vi "Brute Force Measurment SubVI.vi"() -> ()   [LabVIEW 2020]
panel:
  out "Boolean array 2":bool[](array[boolean])
  in  "Number of Active tubes":i32
  out "Clear Pin Task Out 2":refnum<k21>
  in  "Clear Pin Task In 2":refnum<k21>
  in  "Sync Pin Task In":refnum<k21>
  out "Sync Pin Task Out":refnum<k21>
  out "Clear Pin Task Out":refnum<k21>
  in  "Clear Pin Task In":refnum<k21>
  out "Boolean array":bool[](array[boolean])
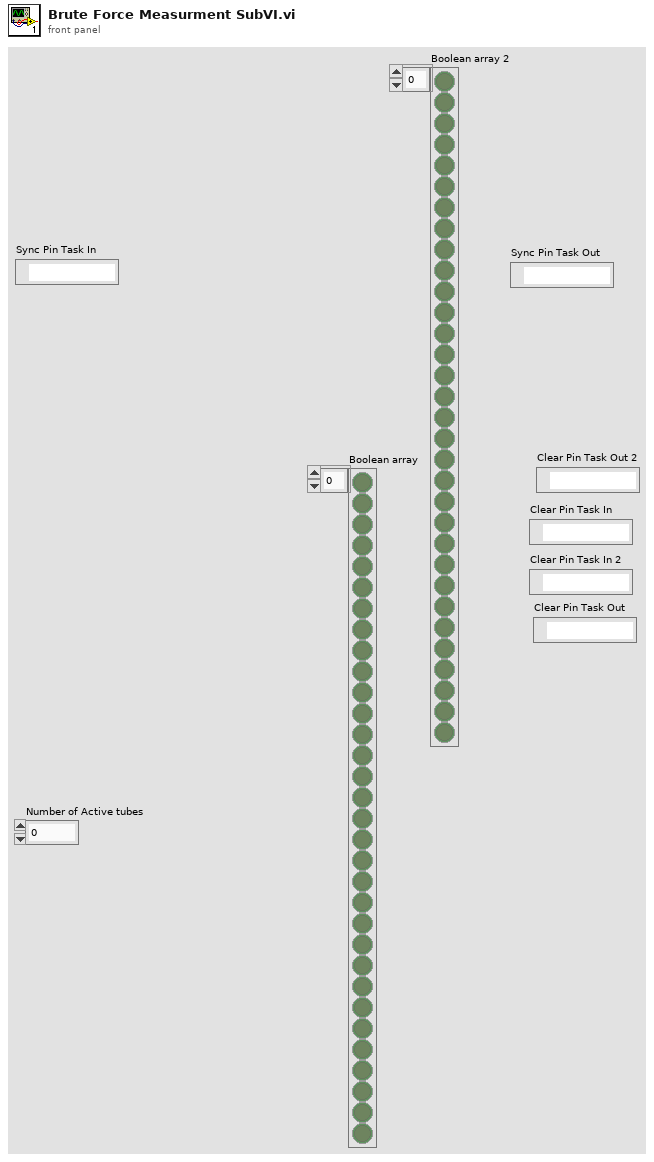
[diagram p1: front panel]
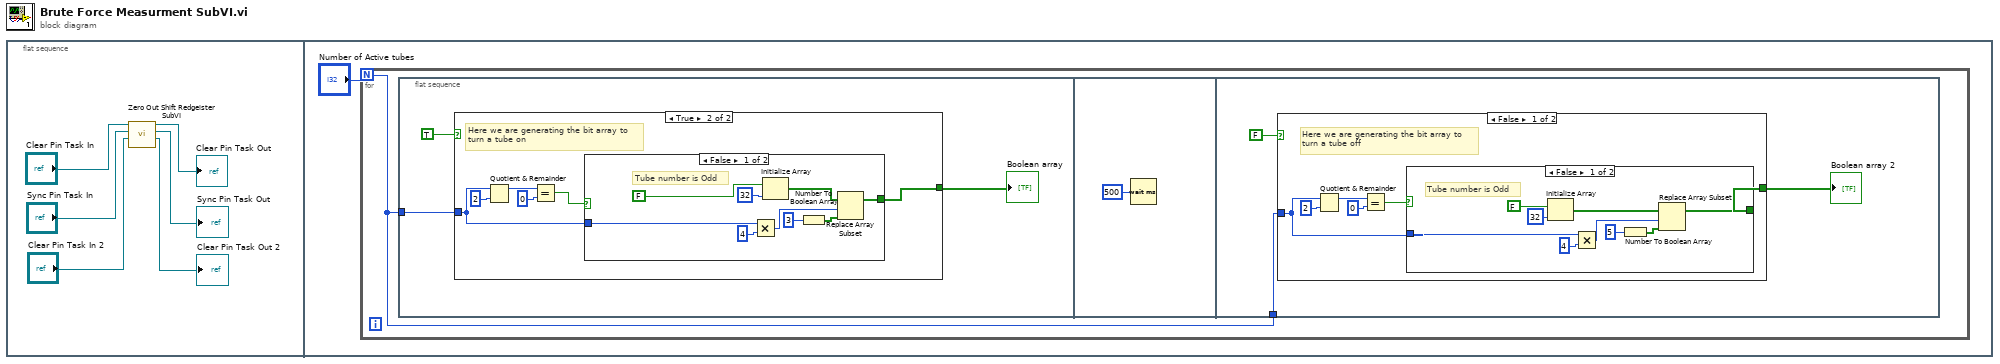
[diagram p0: block diagram]
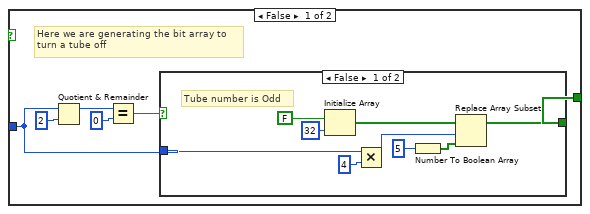
[diagram p2: hidden frame]
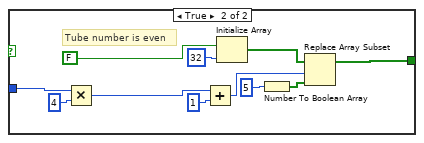
[diagram p3: hidden frame]
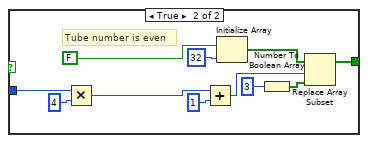
[diagram p4: hidden frame]
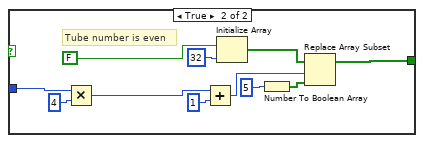
[diagram p5: hidden frame]
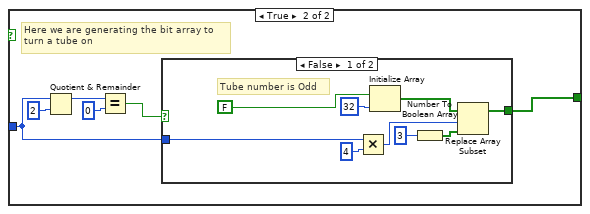
[diagram p6: hidden frame]
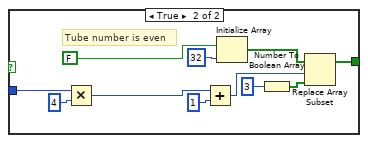
[diagram p7: hidden frame]
diagram:
  n1 = flat-sequence {
    frame #0 {
      n2 = call "Zero Out Shift Redgeister SubVI.vi"("Clear Pin Task In in"="Clear Pin Task In 2", "Sync Pin Task In"="Sync Pin Task In", "Refnum in"="Clear Pin Task In") -> ("Clear Pin Task Out 2"=→"Clear Pin Task Out 2":refnum<k21>, "Sync Pin Task Out"=→"Sync Pin Task Out":refnum<k21>, "Refnum out"=→"Clear Pin Task Out":refnum<k21>)  [unwired: 6 in]
    }
    frame #1 {
      n3 = for {
        N: "Number of Active tubes" -> [w8]
        n4 = flat-sequence {
          tunnel: w8 -> [w10]
          tunnel: w8 -> [w66]
          frame #0 {
            n5 = case shown="True" TRUE {
              tunnel: w10 -> [w13 w42]
              tunnel: [w14 w43] -> w11
              frame False {
                # "Here we are generating the bit array to \nturn a tube off"
                n6 = Quotient & Remainder(x=w13, y=2) -> (x-y*floor(x/y)=w16:i32)  [unwired: 1 out]
                n7 = Equal?(x=w16, y=0) -> (x = y?=w12:bool)
                n8 = case shown="False" w12 {
                  tunnel: w13 -> [w24 w32]
                  tunnel: [w18 w33] -> w14
                  frame False {
                    # "Tube number is Odd"
                    n9 = Initialize Array(FALSE, 32) -> (w20:bool[])
                    n10 = Multiply(x=w24, y=4) -> (x*y=w19:i32)
                    n11 = Number To Boolean Array(number=5) -> (Boolean array=w23:bool[])
                    n12 = Replace Array Subset(array=w20, new element=w23, index=w19) -> (w18:bool[])
                  }
                  frame True {
                    # "Tube number is even"
                    n13 = Multiply(x=w32, y=4) -> (x*y=w28:i32)
                    n14 = Add(x=w28, y=1) -> (x+y=w29:i32)
                    n15 = Initialize Array(FALSE, 32) -> (w35:bool[])
                    n16 = Number To Boolean Array(number=5) -> (Boolean array=w30:bool[])
                    n17 = Replace Array Subset(array=w35, new element=w30, index=w29) -> (w33:bool[])
                  }
                }
              }
              frame True {
                # "Here we are generating the bit array to \nturn a tube on"
                n18 = Quotient & Remainder(x=w42, y=2) -> (x-y*floor(x/y)=w40:i32)  [unwired: 1 out]
                n19 = Equal?(x=w40, y=0) -> (x = y?=w38:bool)
                n20 = case shown="False" w38 {
                  tunnel: w42 -> [w47 w58]
                  tunnel: [w45 w59] -> w43
                  frame False {
                    # "Tube number is Odd"
                    n21 = Multiply(x=w47, y=4) -> (x*y=w46:i32)
                    n22 = Initialize Array(FALSE, 32) -> (w50:bool[])
                    n23 = Number To Boolean Array(number=3) -> (Boolean array=w44:bool[])
                    n24 = Replace Array Subset(array=w50, new element=w44, index=w46) -> (w45:bool[])
                  }
                  frame True {
                    # "Tube number is even"
                    n25 = Multiply(x=w58, y=4) -> (x*y=w54:i32)
                    n26 = Add(x=w54, y=1) -> (x+y=w55:i32)
                    n27 = Initialize Array(FALSE, 32) -> (w61:bool[])
                    n28 = Number To Boolean Array(number=3) -> (Boolean array=w56:bool[])
                    n29 = Replace Array Subset(array=w61, new element=w56, index=w55) -> (w59:bool[])
                  }
                }
              }
            }
            "Boolean array" <- w11
          }
          frame #1 {
            n30 = Wait (ms)(milliseconds to wait=u32 500) -> ()  [unwired: 1 out]
          }
          frame #2 {
            n31 = case shown="False" FALSE {
              tunnel: w66 -> [w69 w98]
              tunnel: [w70 w99] -> w67
              frame False {
                # "Here we are generating the bit array to \nturn a tube off"
                n32 = Quotient & Remainder(x=w69, y=2) -> (x-y*floor(x/y)=w72:i32)  [unwired: 1 out]
                n33 = Equal?(x=w72, y=0) -> (x = y?=w68:bool)
                n34 = case shown="False" w68 {
                  tunnel: w69 -> [w80 w88]
                  tunnel: [w74 w89] -> w70
                  frame False {
                    # "Tube number is Odd"
                    n35 = Initialize Array(FALSE, 32) -> (w76:bool[])
                    n36 = Multiply(x=w80, y=4) -> (x*y=w75:i32)
                    n37 = Number To Boolean Array(number=5) -> (Boolean array=w79:bool[])
                    n38 = Replace Array Subset(array=w76, new element=w79, index=w75) -> (w74:bool[])
                  }
                  frame True {
                    # "Tube number is even"
                    n39 = Multiply(x=w88, y=4) -> (x*y=w84:i32)
                    n40 = Add(x=w84, y=1) -> (x+y=w85:i32)
                    n41 = Initialize Array(FALSE, 32) -> (w91:bool[])
                    n42 = Number To Boolean Array(number=5) -> (Boolean array=w86:bool[])
                    n43 = Replace Array Subset(array=w91, new element=w86, index=w85) -> (w89:bool[])
                  }
                }
              }
              frame True {
                # "Here we are generating the bit array to \nturn a tube on"
                n44 = Quotient & Remainder(x=w98, y=2) -> (x-y*floor(x/y)=w96:i32)  [unwired: 1 out]
                n45 = Equal?(x=w96, y=0) -> (x = y?=w94:bool)
                n46 = case shown="False" w94 {
                  tunnel: w98 -> [w103 w114]
                  tunnel: [w101 w115] -> w99
                  frame False {
                    # "Tube number is Odd"
                    n47 = Multiply(x=w103, y=4) -> (x*y=w102:i32)
                    n48 = Initialize Array(FALSE, 32) -> (w106:bool[])
                    n49 = Number To Boolean Array(number=3) -> (Boolean array=w100:bool[])
                    n50 = Replace Array Subset(array=w106, new element=w100, index=w102) -> (w101:bool[])
                  }
                  frame True {
                    # "Tube number is even"
                    n51 = Multiply(x=w114, y=4) -> (x*y=w110:i32)
                    n52 = Add(x=w110, y=1) -> (x+y=w111:i32)
                    n53 = Initialize Array(FALSE, 32) -> (w117:bool[])
                    n54 = Number To Boolean Array(number=3) -> (Boolean array=w112:bool[])
                    n55 = Replace Array Subset(array=w117, new element=w112, index=w111) -> (w115:bool[])
                  }
                }
              }
            }
            "Boolean array 2" <- w67
          }
        }
      }
    }
  }
